vi "HandleKicker.vi"(10 "cKicker":bool) -> (2 "Output":bool, 3 "Enqueue?":bool)   [LabVIEW 2013]
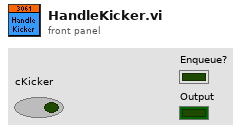
[diagram p1: front panel]
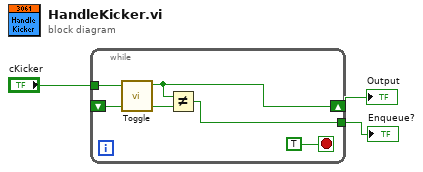
[diagram p0: block diagram]
diagram:
  n1 = while {
    tunnel: "cKicker" -> [w8]
    shift-right: [w7] -> w2
    shift-left: _ -> [w6]
    tunnel: [w5] -> w1
    stop <- TRUE stop-if-true
    n2 = call "Toggle.vi"("Input"=w8) -> ("Output"=w7:bool)  [unwired: 10 in]
    n3 = Not Equal?(x=w7, y=w6) -> (x != y?=w5:bool)
  }
  "Output" <- w2
  "Enqueue?" <- w1
